vi "Acquire.vi"(7 "process name":string, 8 "error in (no error)":errorcluster, 10 "Qbus in":refnum<class "Qbus.lvclass">, 11 "config in":T1) -> (0 "error out":errorcluster, 3 "config out":T1)   [LabVIEW 2017, in "ModbusMaster.lvlib"]
uses:
  <vilib>/addons/InsightCM/Devices/Shared/Common/ModbusMaster/ModbusMaster.lvlib
  <vilib>/addons/InsightCM/Devices/Shared/Common/ModbusMaster/controls/config.ctl
  <vilib>/addons/InsightCM/Devices/Shared/Common/ModbusMaster/controls/ModbusDevice.ctl
  <vilib>/Modbus/master/Modbus Master.lvclass
  <vilib>/addons/InsightCM/Devices/Shared/Common/ModbusMaster/controls/ModbusChannel.ctl
  <vilib>/addons/InsightCM/Devices/Shared/Common/ModbusMaster/controls/RegisterType.ctl
  <vilib>/addons/InsightCM/MessageBus/Base/controls/DataSource.ctl
  <vilib>/addons/InsightCM/MessageBus/Base/controls/KeyValuePair.ctl
  <vilib>/addons/Qbus/Qbus.lvclass
  <vilib>/addons/TimerProcess/controls/taskType.ctl
  <vilib>/addons/TimerProcess/TimerProcess.lvlib
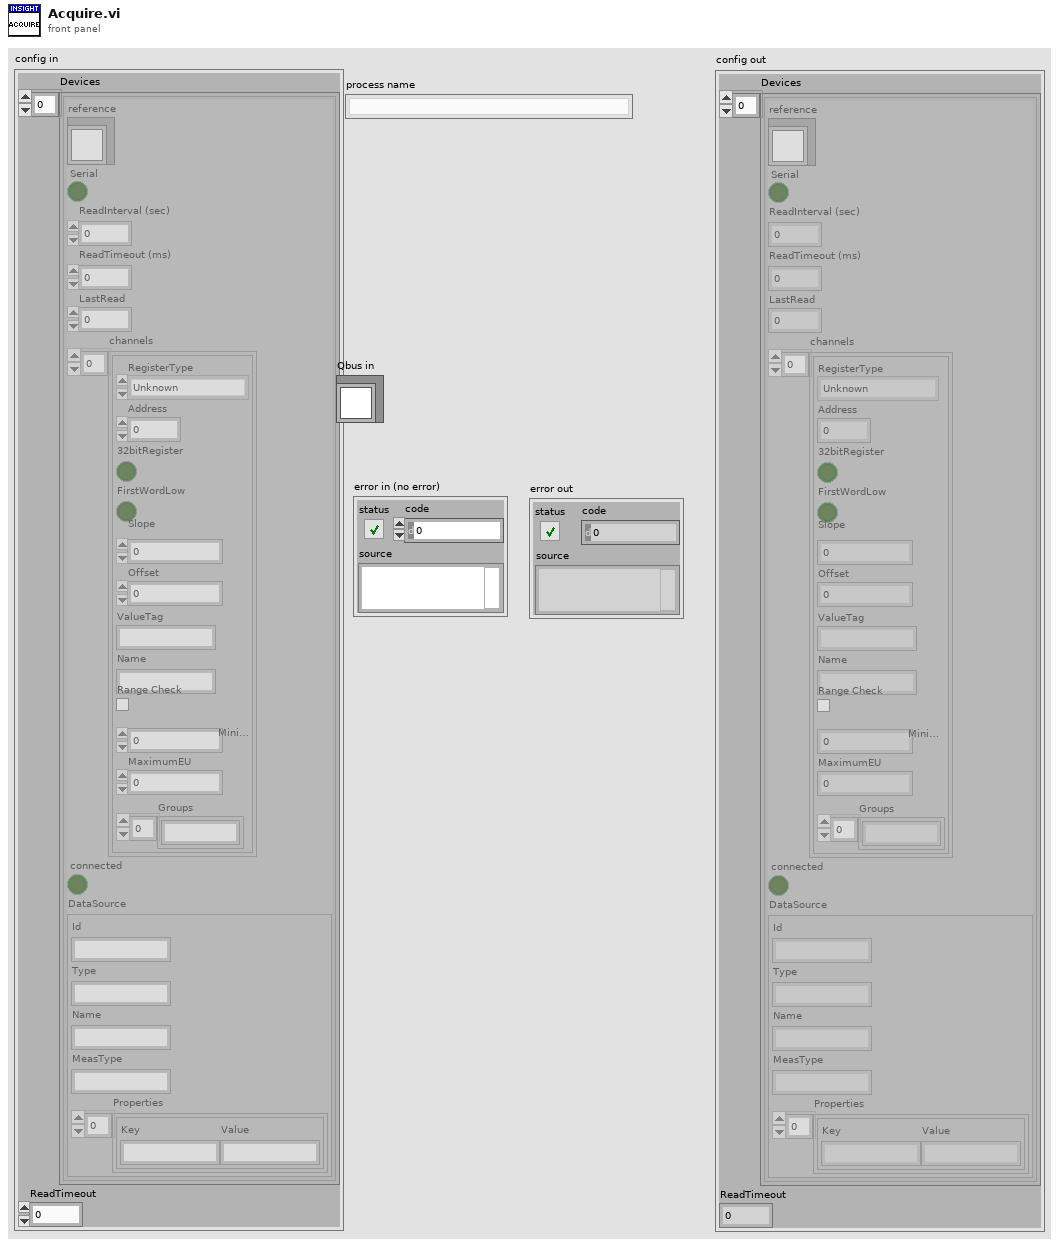
[diagram p1: front panel]
types:
  T1 = typedef "ModbusMaster.lvlib/config.ctl" = cluster{"Devices":T2[], "ReadTimeout":i32}
  T2 = typedef "ModbusMaster.lvlib/ModbusDevice.ctl" = cluster{"reference":refnum<class "Modbus Master.lvclass">, "Serial":bool, "ReadInterval (sec)":dbl, "ReadTimeout (ms)":i32, "LastRead":dbl, "channels":T3[], "connected":bool, "DataSource":T5}
  T3 = typedef "ModbusMaster.lvlib/ModbusChannel.ctl" = cluster{"RegisterType":T4, "Address":i32, "32bitRegister":bool, "FirstWordLow":bool, "Slope":dbl, "Offset":dbl, "ValueTag":string, "Name":string, "Range Check":bool, "MinimumEU":dbl, "MaximumEU":dbl, "Groups":string[]}
  T4 = typedef "ModbusMaster.lvlib/RegisterType.ctl" = enum16{"Unknown", "Coil", "Discrete Input", "Holding Register", "Input Register"}
  T5 = typedef "DataSource.ctl" = cluster{"Id":string, "Type":string, "Name":string, "MeasType":string, "Properties":T6[]}
  T6 = typedef "KeyValuePair.ctl" = cluster{"Key":string, "Value":string}
  T7 = typedef "TimerProcess.lvlib/taskType.ctl" = enum16{"single", "repeat"}
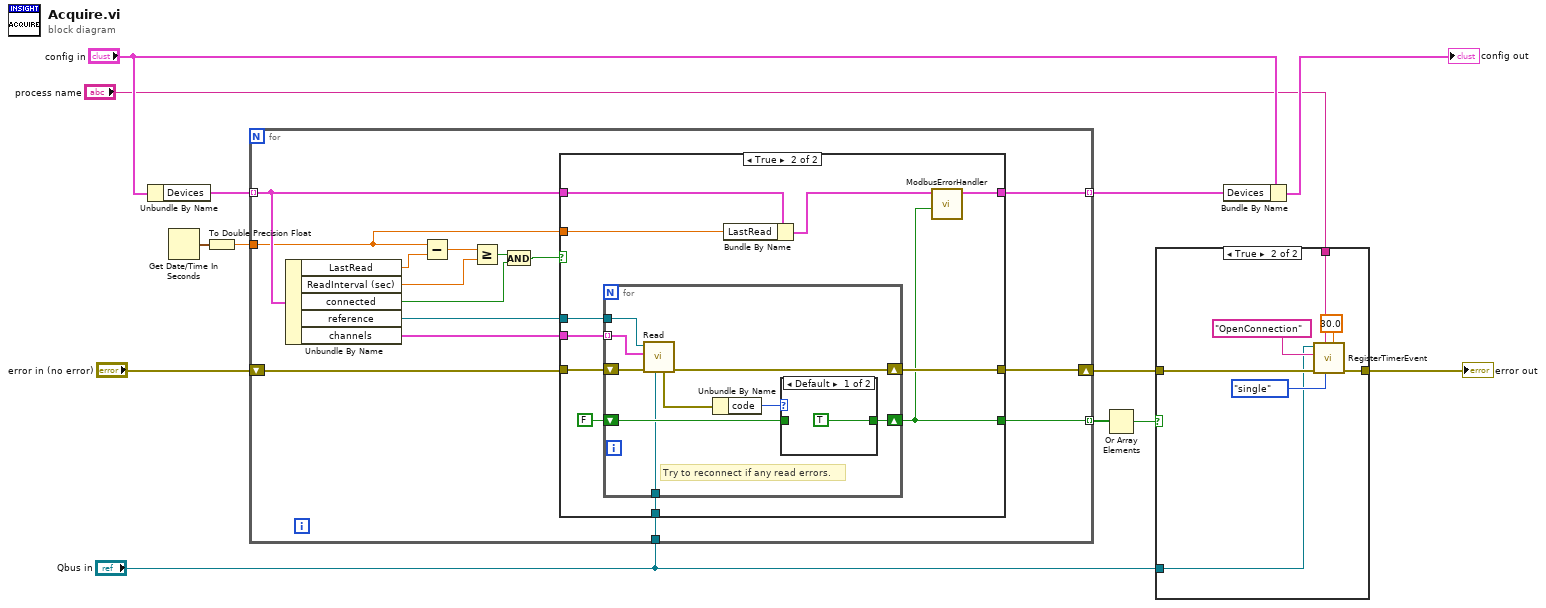
[diagram p0: block diagram]
diagram:
  n1 = Unbundle By Name("config in") -> ("Devices"=w13:T2[])
  n2 = Get Date/Time In Seconds() -> (seconds since 1Jan1904=w9:timestamp)
  n3 = To Double Precision Float(number=w9) -> (double precision float=w8:dbl)
  n4 = for {
    tunnel: w13 -> [w28] mode=indexing
    shift-right: [w27] -> w6
    shift-left: "error in (no error)" -> [w22]
    tunnel: w8 -> [w23]
    tunnel: [w16] -> w7 mode=indexing
    tunnel: [w15] -> w4 mode=indexing
    tunnel: "Qbus in" -> [w14]
    n5 = Unbundle By Name(w28) -> ("LastRead"=w26:dbl, "ReadInterval (sec)"=w24:dbl, "connected"=w17:bool, "reference"=w21:refnum<class "Modbus Master.lvclass">, "channels"=w20:T3[])
    n6 = Subtract(x=w23, y=w26) -> (x-y=w25:dbl)
    n7 = Greater Or Equal?(x=w25, y=w24) -> (x >= y?=w18:bool)
    n8 = And(x=w18, y=w17) -> (x .and. y?=w19:bool)
    n9 = case shown="True" w19 {
      tunnel: w28 -> [w29 w41]
      tunnel: [w30 w36] -> w27
      tunnel: w23 -> [_ w40]
      tunnel: w20 -> [_ w39]
      tunnel: w22 -> [w30 w38]
      tunnel: w21 -> [_ w37]
      tunnel: [w29 w33] -> w16
      tunnel: [_ w32] -> w15
      tunnel: w14 -> [_ w31]
      frame False {
      }
      frame True {
        n10 = for {
          tunnel: w39 -> [w48] mode=indexing
          shift-right: [w47] -> w36
          shift-left: w38 -> [w50]
          tunnel: w37 -> [w49]
          shift-right: [w45] -> w32
          shift-left: FALSE -> [w44]
          tunnel: w31 -> [w42]
          # "Try to reconnect if any read errors."
          n11 = call <vilib>:"Read.vi"("Qbus in"=w42, "error in (no error)"=w50, "channel"=w48, "reference"=w49) -> ("error out"=w47:errorcluster, "read error"=w43:errorcluster)  [unwired: 6 in]
          n12 = Unbundle By Name(w43) -> ("code"=w46:i32)
          n13 = case shown="Default" w46 {
            tunnel: [TRUE w52] -> w45
            tunnel: w44 -> [_ w52]
            frame Default {
            }
            frame 0 {
            }
          }
        }
        n14 = Bundle By Name(cluster=w41, "LastRead"=w40) -> (w34:T2)
        n15 = call <vilib>:"ModbusErrorHandler.vi"("connection error"=w32, "device in"=w34) -> ("device out"=w33:T2)  [unwired: 9 in]
      }
    }
  }
  n16 = Or Array Elements(Boolean array=w4) -> (logical OR=w3:bool)
  n17 = case shown="True" w3 {
    tunnel: w6 -> [w53 w57]
    tunnel: [w53 w56] -> w5
    tunnel: "Qbus in" -> [_ w55]
    tunnel: "process name" -> [_ w54]
    frame False {
    }
    frame True {
      n18 = call <vilib>:"RegisterTimerEvent.vi"("interval (sec)"=30.0, "type"=taskType."single", "process name"=w54, "error in (no error)"=w57, "callback action"="OpenConnection", "qbus in"=w55) -> ("error out"=w56:errorcluster)  [unwired: 4 in, 1 out]
    }
  }
  "error out" <- w5
  n19 = Bundle By Name(cluster="config in", "Devices"=w7) -> (→"config out":T1)
